vi "表达式节点.vi"(10 "华氏温度":dbl) -> (2 "摄氏温度":dbl)   [LabVIEW 2023]
doc: "本VI是为《我和LabVIEW》一书编写的示例。\n关于本书的介绍请参考网页：\nhttp://ruanqizhen.spaces.live.com/blog/cns!5852D4F797C53FB6!4310.entry"
panel:
  out "Numeric":dbl
  out "摄氏温度 2":dbl
  in  "华氏温度 2":dbl
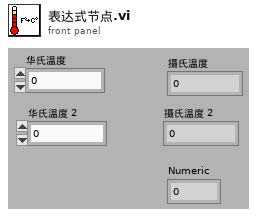
[diagram p1: front panel]
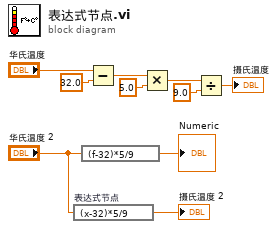
[diagram p0: block diagram]
diagram:
  n1 = expression code="(x-32)*5/9" "表达式节点"("华氏温度 2") -> (→"摄氏温度 2":dbl)
  n2 = expression code="(f-32)*5/9"("华氏温度 2") -> (→"Numeric":dbl)
  n3 = Subtract(x="华氏温度", y=32.0) -> (x-y=w10:dbl)
  n4 = Multiply(x=w10, y=5.0) -> (x*y=w9:dbl)
  n5 = Divide(x=w9, y=9.0) -> (x/y=→"摄氏温度":dbl)
